vi "Nur Zahlen durchlassen.vi"(5 "alte Tabelle":string[][](table), 9 "neue Tabelle":string[][](table), 11 "error in (no error)":errorcluster caption="Fehler (Eingang, kein Fehler)") -> (6 "neue Tabelle":string[][](array[string]), 15 "error out":errorcluster caption="Fehler (Ausgang)")   [LabVIEW 2020, in "Linearisierung v2.lvlib"]
uses:
  Linearisierung v2.lvlib
panel:
  out "Element":bool
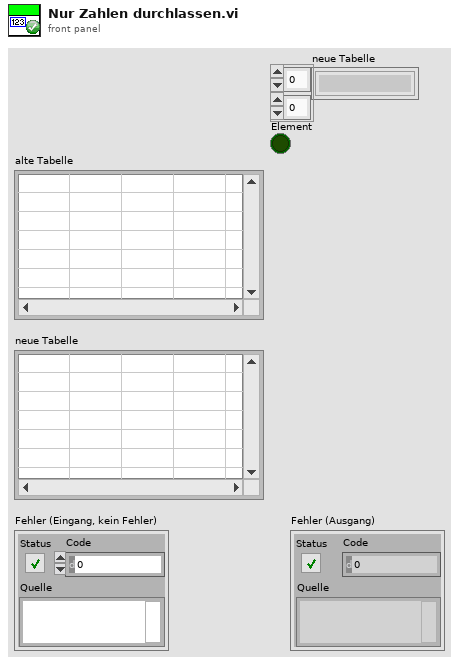
[diagram p1: front panel]
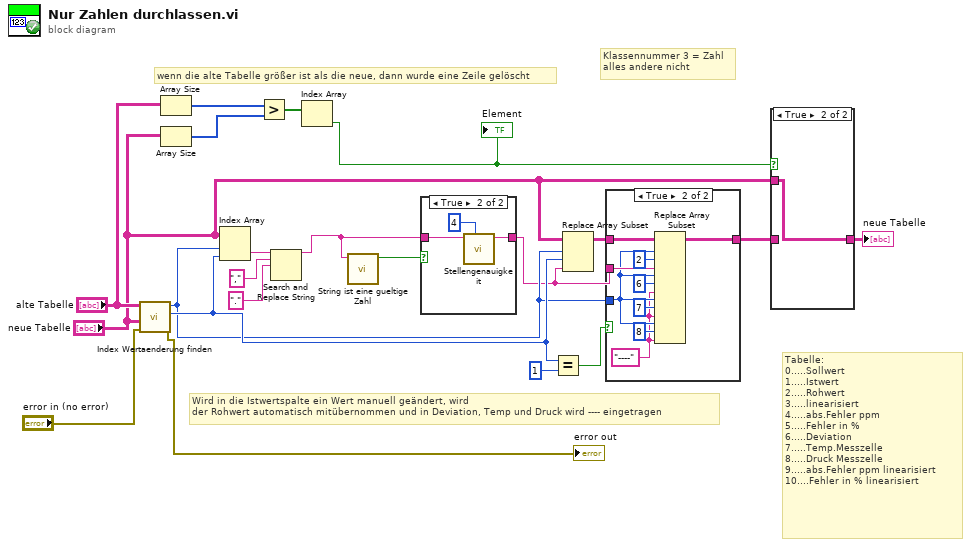
[diagram p0: block diagram]
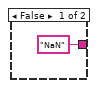
[diagram p4: hidden frame]
diagram:
  # "wenn die alte Tabelle größer ist als die neue, dann wurde eine Zeile gelöscht"
  # "Tabelle:\n0.....Sollwert\n1.....Istwert\n2.....Rohwert\n3.....linearisiert\n4.....abs.Fehler ppm\n5.....Fehler in %\n6.....Deviation\n7.....Temp.Messzelle\n8.....Druck Messzelle\n9.....abs.Fehler ppm linearisiert\n10....Fehler in % linearisiert"
  # "Wird in die Istwertspalte ein Wert manuell geändert, wird \nder Rohwert automatisch mitübernommen und in Deviation, Temp und Druck wird ---- eingetragen"
  # "Klassennummer 3 = Zahl\nalles andere nicht"
  n1 = call "Index Wertaenderung finden.vi"("error in (no error)"="error in (no error)", "neue Tabelle"="neue Tabelle", "alte Tabelle"="alte Tabelle") -> ("error out"=→"error out":errorcluster, "Spalte"=w13:i32, "Zeile"=w10:i32)  [unwired: 6 in]
  n2 = Array Size(array="alte Tabelle") -> (size(s)=w5:i32[])
  n3 = Array Size(array="neue Tabelle") -> (size(s)=w4:i32[])
  n4 = Index Array(array="neue Tabelle", index (row)=w10, index (col)=w13) -> (element=w19:string)
  n5 = Greater?(x=w5, y=w4) -> (0:w3:bool[])
  n6 = Search and Replace String(input string=w19, search string="," ("Such-String"), replace string="." ("Ersetzungs-String (\"\")")) -> (result string=w18:string)  [unwired: 5 in, 3 out]
  n7 = Index Array(array=w3) -> (element=w2:bool)  [unwired: 1 in]
  "Element" <- w2
  n8 = call "String ist eine gueltige Zahl.vi"("String"=w18) -> ("Zahl"=w17:bool)  [unwired: 10 in]
  n9 = case shown="True" w17 {
    tunnel: w18 -> [_ w25]
    tunnel: ["NaN" ("result string") w24] -> w9
    frame False {
    }
    frame True {
      n10 = call "Stellengenauigkeit.vi"("Genauigkeit (6)"=i16 4, "String"=w25) -> ("String out"=w24:string)  [unwired: 8 in, 1 out]
    }
  }
  n11 = Equal?(x=w13, y=1) -> (x = y?=w11:bool)
  n12 = Replace Array Subset(array="neue Tabelle", new element=w9, index (row)=w10, index (col)=w13) -> (w14:string[][])
  n13 = case shown="True" w11 {
    tunnel: w14 -> [w26 w35]
    tunnel: [w26 w34] -> w7
    tunnel: w10 -> [_ w31]
    tunnel: w9 -> [_ w32]
    frame False {
    }
    frame True {
      w27 = "----" ("Neues Element/Teil-Array")
      n14 = Replace Array Subset(array=w35, new element #1=w32, index (row) #1=w31, index (col) #1=2 ("Deaktivierter Index (Spalte)"), new element #2=w27, index (row) #2=w31, index (col) #2=6 ("Deaktivierter Index (Spalte)"), new element #3=w27, index (row) #3=w31, index (col) #3=7 ("Deaktivierter Index (Spalte)"), new element #4=w27, index (row) #4=w31, index (col) #4=8 ("Deaktivierter Index (Spalte)")) -> (w34:string[][])
    }
  }
  n15 = case shown="True" w2 {
    tunnel: w7 -> [w36 _]
    tunnel: [w36 w37] -> w6
    tunnel: "neue Tabelle" -> [_ w37]
    frame False {
    }
    frame True {
    }
  }
  "neue Tabelle" <- w6
